vi "Convert to String.vi"(10 "byte array":u8[](array[numeric]), 11 "number of objects":u8) -> (3 "objects":cluster{"object ID":u8, "value":string}[](array[cluster]) {"object ID" format="%x"})   [LabVIEW 2020, in "SubVIs.lvlib" / "Master Function Definition.lvlib"]
uses:
  <vilib>/Modbus/subvis/Data and Functions/Master Function Definition/Master Function Definition.lvlib
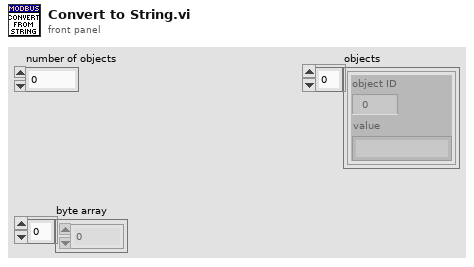
[diagram p1: front panel]
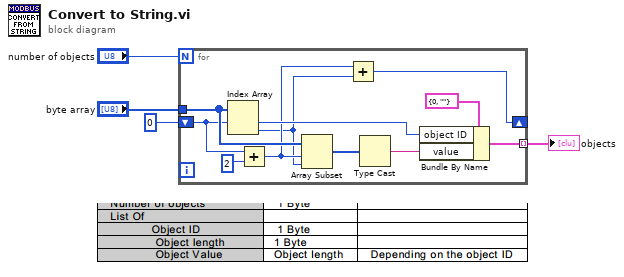
[diagram p0: block diagram]
diagram:
  n1 = for {
    N: "number of objects" -> [_]
    shift-right: [w6] -> _
    shift-left: 0 -> [w9]
    tunnel: [w14] -> w1 mode=indexing
    tunnel: "byte array" -> [w11]
    n2 = Index Array(array=w11, index #1=w9) -> (element #1=w12:u8, element #2=w5:u8)  [unwired: 1 in]
    n3 = Add(x=w9, y=2) -> (x+y=w7:i32)
    n4 = Array Subset(array=w11, index=w7, length=w5) -> (w10:u8[])
    n5 = Add(x=w7, y=w5) -> (x+y=w6:i32)
    n6 = Type Cast(x=w10) -> (*(type *) &x=w13:string)  [unwired: 1 in]
    n7 = Bundle By Name(cluster=cluster{"object ID":u8, "value":string} {"object ID"=0, "value"=""} ("Cluster"), "object ID"=w12, "value"=w13) -> (w14:cluster{"object ID":u8, "value":string})
  }
  "objects" <- w1
